vi "Finish.vi"   [LabVIEW 2015]
doc: "This VI is called just before exiting. It is expected to close I/O refnum, save collected data, etc."
uses:
  Refname/Refname Enum (Queue).ctl
  Refname/Refname Enum (Joystick).ctl
  Refname/Refname Enum (Actuator).ctl
  Refname/Refname to String (Actuator).vi
  Refname/Refname to String (Joystick).vi
  Refname/Refname to String (Queue).vi
  <vilib>/Rock Robotics/WPI/Utilities/WPI_GetSetVariantRefNum.vi
  lib/Sprocket.lvlib
types:
  T1 = typedef "Sprocket.lvlib/Refname Enum (Actuator).ctl" = enum16{"Drive Motors"}
  T2 = typedef "Sprocket.lvlib/Refname Enum (Joystick).ctl" = enum16{"Joystick 0", "Joystick 1", "Joystick 2", "Joystick 3"}
  T3 = typedef "Sprocket.lvlib/Refname Enum (Queue).ctl" = enum16{"Input", "Drive"}
  T4 = typedef "WPI_JoystickDevRef.ctl" = cluster{"Device":T5}
  T5 = typedef "WPI_JoystickDeviceEnum.ctl" = enum16{"USB 0", "USB 1", "USB 2", "USB 3", "USB 4", "USB 5"}
  T6 = typedef "WPI_RobotDriveDevRef.ctl" = cluster{"DevStatus":errorcluster, "Motors[]":T7[], "Square Inputs":bool, "Max Output":dbl}
  T7 = typedef "WPI_MotorControlDeviceRef.ctl" = cluster{"DeviceStatus":errorcluster, "Type":T8, "PWM":cluster{"PWM Channel":T9, "DeadBand":T10}, "CAN":cluster{"Device Number":u8, "Control Mode":T11, "Semaphore":T12, "Max Vout":dbl, "TalonSRX Control Mode":T13}, "Invert":bool}
  T8 = typedef "WPI_MotorControlType.ctl" = enum16{"PWM", "CAN", "CANTalonSRX"}
  T9 = typedef "FPGA_DIOPWMChannel.ctl" = enum8{"PWM 0", "PWM 1", "PWM 2", "PWM 3", "PWM 4", "PWM 5", "PWM 6", "PWM 7", "PWM 8", "PWM 9", "PWM MXP 0", "PWM MXP 1", "PWM MXP 2", "PWM MXP 3", "PWM MXP 4", "PWM MXP 5", "PWM MXP 6", "PWM MXP 7", "PWM MXP 8", "PWM MXP 9", "Invalid"}
  T10 = typedef "WPI_PWMDeadband.ctl" = cluster{"Name":string, "maxPositivePwm":i32, "minPositivePwm":i32, "centerPwm":i32, "maxNegativePwm":i32, "minNegativePwm":i32, "angularRange":u16}
  T11 = typedef "WPI_CANJaguar_ControlMode.ctl" = enum8{"Percent VBus", "Current", "Speed", "Position", "Voltage"}
  T12 = typedef "Semaphore RefNum" = refnum<k1>
  T13 = typedef "WPI_CANTalonSRX_APIControlMode.ctl" = enum8{"Percent VBus", "Speed", "Position", "Slave", "Unchanged / Invalid", "Voltage Compensation", "Current", "Motion Profile"}
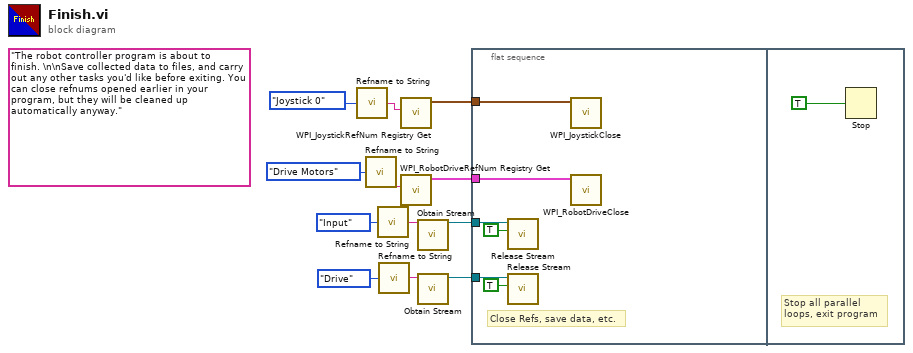
[diagram p0: block diagram]
diagram:
  (unwired) "The robot controller program is about to finish. \n\nSave collected data to files, and carry out any other tasks you'd like before exiting. You can close refnums opened earlier in your program, but they will be cleaned up automatically anyway."
  n1 = call-poly "Refname to String.vi"("Joystick Refname"=Refname_Enum_(Joystick)."Joystick 0") -> ("Refnum Name"=w5:string)
  n2 = call-poly "Refname to String.vi"("Actuator Refname"=Refname_Enum_(Actuator)."Drive Motors") -> ("Refnum Name"=w2:string)
  n3 = call-poly "Refname to String.vi"("Queue Refname"=Refname_Enum_(Queue)."Input" ("Refname (Queue)")) -> ("Refnum Name"=w9:string)
  n4 = call-poly "Refname to String.vi"("Queue Refname"=Refname_Enum_(Queue)."Drive" ("Refname (Queue)")) -> ("Refnum Name"=w8:string)
  n5 = call <vilib>:"WPI_JoystickRefNum Registry Get.vi"("refnum name"=w5) -> ("JoystickDevRef"=w11:T4)  [unwired: 1 in, 9 out]
  n6 = call <vilib>:"WPI_RobotDriveRefNum Registry Get.vi"("refnum name"=w2) -> ("RobotDriveDevRef"=w12:T6)  [unwired: 1 in, 9 out]
  n7 = call "Obtain Stream.vi"("Name"=w9) -> ("stream out"=w4:refnum<queue>)  [unwired: 9 in, 1 out]
  n8 = call "Obtain Stream.vi"("Name"=w8) -> ("stream out"=w3:refnum<queue>)  [unwired: 9 in, 1 out]
  n9 = flat-sequence {
    tunnel: w12 -> [w18]
    tunnel: w11 -> [w17]
    tunnel: w4 -> [w16]
    tunnel: w3 -> [w15]
    frame #0 {
      # "Close Refs, save data, etc."
      n10 = call "Release Stream.vi"("force destroy? (F)"=TRUE, "stream in"=w16) -> ()  [unwired: 8 in, 2 out]
      n11 = call "Release Stream.vi"("force destroy? (F)"=TRUE, "stream in"=w15) -> ()  [unwired: 8 in, 2 out]
      n12 = call <vilib>:"WPI_JoystickClose.vi"("JoystickDevRef"=w17) -> ()  [unwired: 11 out]
      n13 = call <vilib>:"WPI_RobotDriveClose.vi"("RobotDriveDevRef"=w18) -> ()  [unwired: 1 in, 10 out]
    }
    frame #1 {
      # "Stop all parallel\nloops, exit program"
      n14 = Stop(stop? (T)=TRUE ("Quit")) -> ()
    }
  }
